vi "GenerateUpcomingReport.vi"() -> ()   [LabVIEW 2024]
uses:
  TypeDefs/comics.reply--cluster.ctl
  TypeDefs/comic--cluster.ctl
  <vilib>/addons/_JKI.lib/Serialization/JSON/JKI JSON Serialization.lvlib
  <userlib>/_OpenG.lib/string/string.llb/openg_string.lvlib
panel:
  out "title out":string
  out "delimited string":string
  out "error out":errorcluster
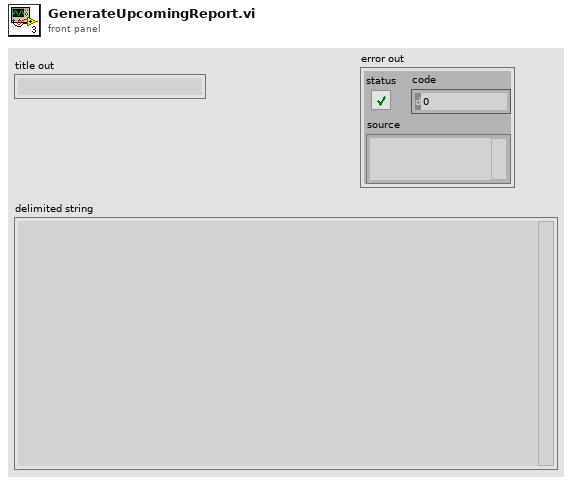
[diagram p1: front panel]
types:
  T1 = typedef "comics.reply--cluster.ctl" = cluster{"code":i32, "status":string, "etag":string, "data":cluster{"offset":i32, "limit":i32, "total":i32, "count":i32, "results":T2[]}}
  T2 = typedef "comic--cluster.ctl" = cluster{"id":i32, "digitalId":i32, "title":string, "issueNumber":i32, "variantDescription":string, "description":string, "modified":variant, "upc":string, "format":string, "pageCount":i32, "resourceURI":string, "urls":cluster{"type":string, "url":string}[], "series":cluster{"resourceURI":string, "name":string}, "dates":cluster{"type":string, "date":string}[], "prices":cluster{"price":dbl, "type":string}[], "thumbnail":cluster{"path":string, "extension":string}, "images":cluster{"path":string, "extension":string}[], "creators":cluster{"available":i32, "returned":i32, "collectionURI":string, "items":cluster{"resourceURI":string, "name":string, "role":string}[]}, "characters":cluster{"available":i32, "returned":i32, "collectionURI":string, "items":cluster{"resourceURI":string, "name":string}[]}, "stories":cluster{"available":i32, "returned":i32, "collectionURI":string, "items":cluster{"resourceURI":string, "name":string, "type":string}[]}, "events":cluster{"available":i32, "returned":i32, "collectionURI":string, "items":cluster{"resourceURI":string, "name":string}[]}}
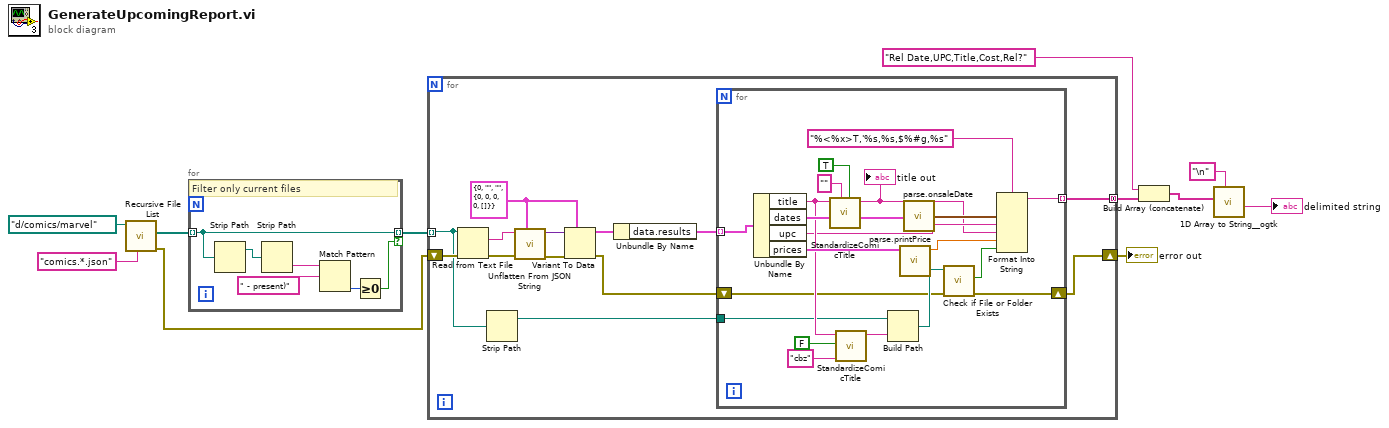
[diagram p0: block diagram]
diagram:
  n1 = call <vilib>:"Recursive File List.vi"("pattern"="comics.*.json", "Folder Path"=path "d:/comics/marvel") -> ("error out"=w7:errorcluster, "All Files in Dir"=w9:path[])  [unwired: 5 in, 3 out]
  n2 = for {
    tunnel: w9 -> [w13] mode=indexing
    tunnel: [w13] -> w8 mode=indexing if=w12
    # "Filter only current files"
    n3 = Strip Path(path=w13) -> (stripped path=w17:path)  [unwired: 1 out]
    n4 = Strip Path(path=w17) -> (name=w16:string)  [unwired: 1 out]
    n5 = Match Pattern(string=w16, regular expression=" - present)") -> (offset past match=w14:i32)  [unwired: 1 in, 3 out]
    n6 = Greater Or Equal To 0?(x=w14) -> (x >= 0?=w12:bool)
  }
  n7 = for {
    tunnel: w8 -> [w22] mode=indexing
    shift-right: [w19] -> w6
    shift-left: w7 -> [w30]
    tunnel: [w18] -> w3 mode=concatenating
    w25 = T1 {"code"=0, "status"="", "etag"="", "data"={"offset"=0, "limit"=0, "total"=0, "count"=0, "results"=[]}} ("reply")
    n8 = Read from Text File(file (use dialog)=w22, error in=w30) -> (text=w28:string, error out=w29:errorcluster)  [unwired: 2 in, 2 out]
    n9 = Strip Path(path=w22) -> (stripped path=w21:path)  [unwired: 1 out]
    n10 = call <vilib>:"Unflatten From JSON String.vi"("Type and Defaults"=w25, "error in (no error)"=w29, "JSON String"=w28) -> ("error out"=w27:errorcluster, "Variant"=w26:variant)  [unwired: 7 in]
    n11 = Variant To Data(error in=w27, type=w25, Variant=w26) -> (data=w24:T1, error out=w20:errorcluster)
    n12 = Unbundle By Name(w24) -> ("data.results"=w23:T2[])
    n13 = for {
      tunnel: w23 -> [w50] mode=indexing
      tunnel: w21 -> [w42]
      shift-right: [w33] -> w19
      shift-left: w20 -> [w34]
      tunnel: [w32] -> w18 mode=indexing
      n14 = Unbundle By Name(w50) -> ("title"=w46:string, "dates"=w48:cluster{"type":string, "date":string}[], "upc"=w38:string, "prices"=w47:cluster{"price":dbl, "type":string}[])
      n15 = call "StandardizeComicTitle.vi"("make sortable (F)"=TRUE, "extention (\"\"=none)"="" ("extention (\"\"=none)"), "title in"=w46) -> ("title out"=w37:string)  [unwired: 8 in]
      "title out" <- w37
      n16 = call "StandardizeComicTitle.vi"("make sortable (F)"=FALSE, "extention (\"\"=none)"="cbz" ("extention (\"\"=none)"), "title in"=w46) -> ("title out"=w43:string)  [unwired: 8 in]
      n17 = Build Path(base path=w42, name or relative path=w43) -> (appended path=w41:path)
      n18 = call "parse.printPrice.vi"("prices"=w47) -> ("price"=w36:sgl)  [unwired: 6 in]
      n19 = call "parse.onsaleDate.vi"("dates"=w48) -> ("Time Stamp"=w39:timestamp)
      n20 = call <vilib>:"Check if File or Folder Exists.vi"("error in (no error)"=w34, "path"=w41) -> ("error out"=w33:errorcluster, "file or folder exists?"=w35:bool)  [unwired: 7 in, 1 out]
      n21 = Format Into String(format string="%<%x>T,'%s,%s,$%#g,%s", w39, w38, w37, w36, w35) -> (resulting string=w32:string)  [unwired: 2 in, 1 out]
    }
  }
  "error out" <- w6
  n22 = Build Array (concatenate)("Rel Date,UPC,Title,Cost,Rel?", w3) -> (w1:string[])
  n23 = call <userlib>:"1D Array to String__ogtk.vi"("delimiter (Tab)"="\n", "Array of Strings"=w1) -> ("delimited string"=→"delimited string":string)  [unwired: 9 in]
